vi "Error_Handler_MHL_FGV.vi"(6 "Exit on Error? (F)":bool, 7 "Case":string, 8 "error in (no error)":errorcluster, 9 "VI_name":string, 10 "queue IN":refnum<queue>, 11 "Ignore Errors (Runtime)":i32[](array[numeric])) -> (0 "error Out":errorcluster)   [LabVIEW 2024, in "Relay_Module.lvlib"]
doc: "This VI\n---------------------------------------------------------\nMessage_Loop_Handler_FGV.\n---------------------------------------------------------\n-Handels the error occured in message handling loop"
uses:
  Relay_Module.lvlib
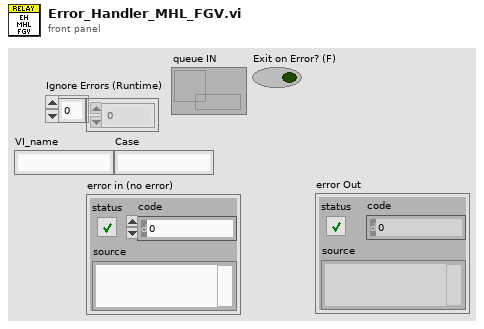
[diagram p1: front panel]
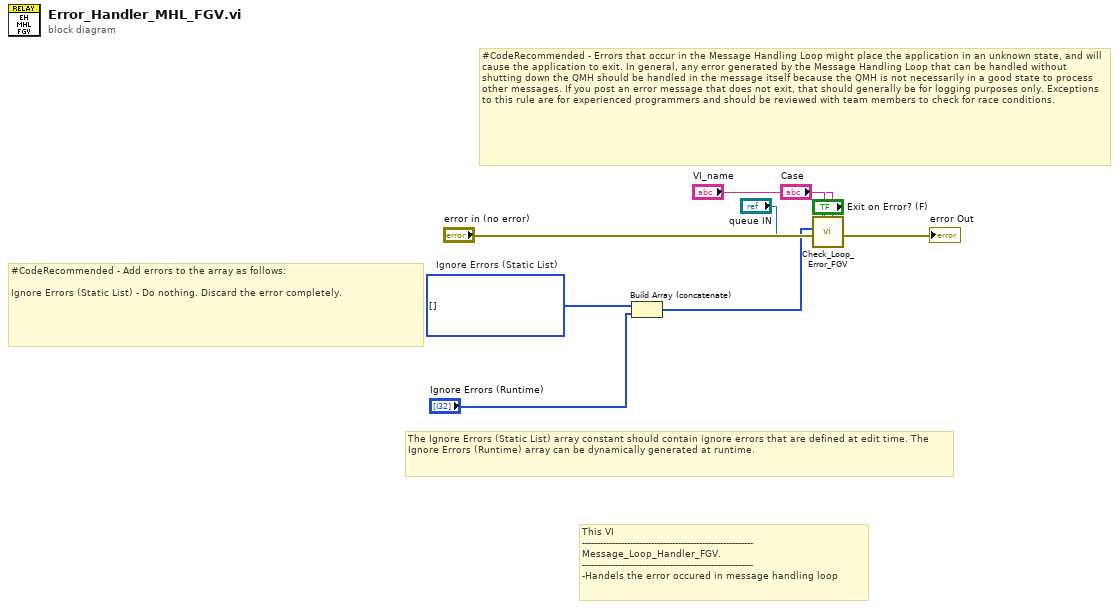
[diagram p0: block diagram]
diagram:
  w4 = i32[] []  # Ignore Errors (Static List)
  # "This VI\n---------------------------------------------------------\nMessage_Loop_Handler_FGV.\n---------------------------------------------------------\n-Handels the error occured in message handling loop"
  # "#CodeRecommended - Errors that occur in the Message Handling Loop might place the application in an unknown state, and will cause the application to exit. In general, any error generated by the Message Handling Loop that can be handled without shutting down the QMH should be handled in the message itself because the QMH is not necessarily in a good state to process other messages. If you post an error message that does not exit, that should generally be for logging purposes only. Exceptions to this rule are for experienced programmers and should be reviewed with team members to check for race conditions."
  # "The Ignore Errors (Static List) array constant should contain ignore errors that are defined at edit time. The Ignore Errors (Runtime) array can be dynamically generated at runtime."
  # "#CodeRecommended - Add errors to the array as follows:\n\nIgnore Errors (Static List) - Do nothing. Discard the error completely."
  n1 = Build Array (concatenate)(w4, "Ignore Errors (Runtime)") -> (w7:i32[])
  n2 = call "Check_Loop_Error_FGV.vi"("Case"="Case", "VI_name"="VI_name", "error in (no error)"="error in (no error)", "queue IN"="queue IN", "Ignore Errors"=w7, "Exit on Error? (F)"="Exit on Error? (F)") -> ()  [unwired: 5 in, 1 out]
  "error Out" <- "error in (no error)"
